vi "Write Configuration File.vi"(8 "error in (no error)":errorcluster, 11 "Sequence Experiment":refnum<class "Control Experiment.lvclass">) -> (0 "error out":errorcluster, 3 "Sequence Experiment out":refnum<class "Control Experiment.lvclass">)   [LabVIEW 2016, in "Control Experiment.lvclass"]
uses:
  Control Experiment.lvclass
  C:/Program Files (x86)/National Instruments/LabVIEW 2016/user.lib/LevyLab/Levylab Instruments/SMOs/Instrument/Instrument.lvclass
  <userlib>/LevyLab/Levylab Instruments/SMOs/Instrument/Instrument.lvclass/Instrument.ctl
  Control Experiment.lvclass/Control Experiment.ctl
  <userlib>/LevyLab/Levylab Instruments/SMOs/Configuration/Configuration.lvclass
  <userlib>/LevyLab/Levylab Instruments/SMOs/Instrument/Instrument.lvclass
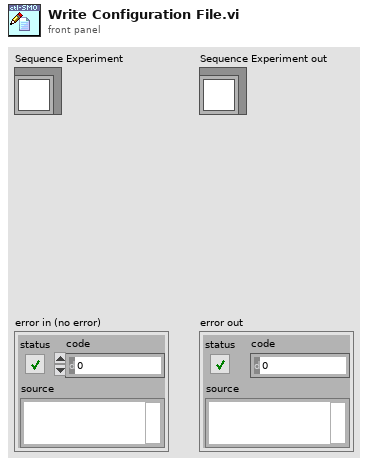
[diagram p1: front panel]
types:
  T1 = typedef "Control Experiment.lvclass/Control Experiment.Configuration--Cluster.ctl" = cluster{"Example Setting 1":dbl, "Example Setting 2":dbl, "Example Setting 3":string}
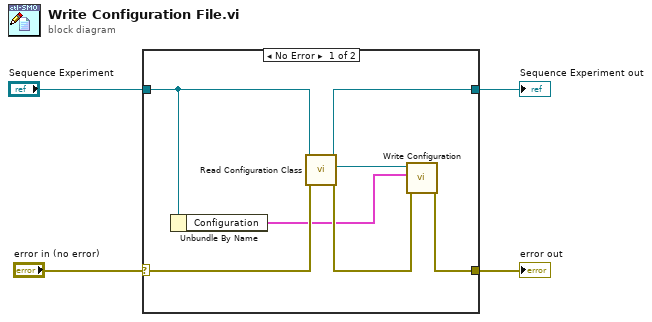
[diagram p0: block diagram]
diagram:
  n1 = case shown="No Error" "error in (no error)" {
    selector: "error in (no error)" -> [w7 w13]
    tunnel: "Sequence Experiment" -> [w6 w12]
    tunnel: [w10 w12] -> w3
    tunnel: [w9 w13] -> w2
    frame No Error {
      n2 = Unbundle By Name(w6) -> ("Configuration"=w5:T1)
      n3 = call <userlib>:"Read Configuration Class.vi"("error in (no error)"=w7, "Instrument in"=w6) -> ("error out"=w11:errorcluster, "Configuration.lvclass"=w8:refnum<class "Configuration.lvclass">, "Instrument out"=w10:refnum<class "Control Experiment.lvclass">)  [unwired: 7 in]
      n4 = call <userlib>:"Write Configuration.vi"("error in (no error)"=w11, "Variant"=w5, "Configuration in"=w8) -> ("error out"=w9:errorcluster)  [unwired: 7 in, 1 out]
    }
    frame Error {
    }
  }
  "Sequence Experiment out" <- w3
  "error out" <- w2
